vi "PIDController_AdvCalculate_FF_Sp_Pv.vi"(6 "Time":dbl=-1.0 format="%33.4f", 7 "Auto":bool=TRUE, 8 "FF":dbl, 9 "SP":dbl, 10 "PV":dbl, 11 "in PID_CONTROLLER":T1={"Kp"=0.0, "Ki"=0.0, "Kd"=0.0, "Period"=0.0, "Max_Integral"=0.0, "Min_Integral"=0.0, "Max_Input"=0.0, "Min_Input"=0.0, "Continuous"=FALSE, "PositionError"=0.0, "VelocityError"=0.0, "PrevError"=0.0, "TotalError"=0.0, "PositionTolerance"=0.0, "VelocityTolerance"=0.0, "SetPoint"=0.0, "Kf"=0.0, "Prev_Deriv"=0.0, "Prev_Deriv 2"=0.0, "DerivativeFilter"=FALSE, "Min_Output"=-9.99e+35, "Max_Output"=9.9e+35, "Prev_F_P"=0.0, "Prev_F_P_2"=0.0, "AntiWindupActive"=FALSE, "Measurement"=0.0} {"Measurement" format="%16_6e"; "Prev_F_P_2" format="%16_6e"; "Prev_F_P" format="%16_6e"; "Max_Output" format="%16_6e"; "Min_Output" format="%16_6e"; "Prev_Deriv 2" format="%16_6e"; "Prev_Deriv" format="%16_6e"; "Kf" format="%16_6e"; "SetPoint" format="%16_6e"; "VelocityTolerance" format="%16_6e"; "PositionTolerance" format="%16_6e"; "TotalError" format="%16_6e"; "PrevError" format="%16_6e"; "VelocityError" format="%16_6e"; "PositionError" format="%16_6e"; "Min_Input" format="%16_6e"; "Max_Input" format="%16_6e"; "Min_Integral" format="%16_6e"; "Max_Integral" format="%16_6e"; "Period" format="%16_6e"; "Kd" format="%16_6e"; "Ki" format="%16_6e"; "Kp" format="%16_6e"}) -> (1 "ControlOutput":dbl, 3 "out PID_CONTROLLER":T1={"Kp"=0.0, "Ki"=0.0, "Kd"=0.0, "Period"=0.0, "Max_Integral"=0.0, "Min_Integral"=0.0, "Max_Input"=0.0, "Min_Input"=0.0, "Continuous"=FALSE, "PositionError"=0.0, "VelocityError"=0.0, "PrevError"=0.0, "TotalError"=0.0, "PositionTolerance"=0.0, "VelocityTolerance"=0.0, "SetPoint"=0.0, "Kf"=0.0, "Prev_Deriv"=0.0, "Prev_Deriv 2"=0.0, "DerivativeFilter"=FALSE, "Min_Output"=-9.99e+35, "Max_Output"=9.9e+35, "Prev_F_P"=0.0, "Prev_F_P_2"=0.0, "AntiWindupActive"=FALSE, "Measurement"=0.0} {"Measurement" format="%16_6e"; "Prev_F_P_2" format="%16_6e"; "Prev_F_P" format="%16_6e"; "Max_Output" format="%16_6e"; "Min_Output" format="%16_6e"; "Prev_Deriv 2" format="%16_6e"; "Prev_Deriv" format="%16_6e"; "Kf" format="%16_6e"; "SetPoint" format="%16_6e"; "VelocityTolerance" format="%16_6e"; "PositionTolerance" format="%16_6e"; "TotalError" format="%16_6e"; "PrevError" format="%16_6e"; "VelocityError" format="%16_6e"; "PositionError" format="%16_6e"; "Min_Input" format="%16_6e"; "Max_Input" format="%16_6e"; "Min_Integral" format="%16_6e"; "Max_Integral" format="%16_6e"; "Period" format="%16_6e"; "Kd" format="%16_6e"; "Ki" format="%16_6e"; "Kp" format="%16_6e"})   [LabVIEW 2019, in "Trajectory_Library.lvlib"]
doc: "Returns the next output of the \"advanced\" PID controller. This controller implements the same PID as the \"normal\" controller with the following enhancements:\n - Integration by trapezoids is used.\n - Optionally filters derivative terms. (See SetDerivativeFilter subVI documentation for information.)\n - Incorporates optional feedforward.\n - Includes integral windup protection. This is only useful when output limits are specified.\n - When not called with a specific period, uses the actual elapsed time. (This subVI calculates the actual elapsed time.) \n - Limits the outputs. When output limits are specified the output is cooerced be within these limits.\n - Includes an Auto/Manual mode. In manual mode the scaled feedforward is sent directly to the output and the PID controller tracks this output value to allow for smooth transition back to auto mode.\n\nThe generalized equation for this PID when in auto is:\n CO = Kf x feedforward + Kp x error + Ki x Integral(error) + Kd x Derivative(error)\n\nWhen auto mode is disabled, the generaized equation is:\n CO = Kf x feedforward \n \nInputs:\n - PID_Controller -- PID_Controller data cluster\n - PV-measurement -- The current measurement of the process variable. (PV)\n - SP-setpoint -- The new setpoint of the controller. (SP)\n - FF-feedforward -- Feedforward n the same units as the PV and SP\n - Auto -- Use the PID calculate when this is True\n\nOutputs:\n - PID_Controller -- Updated PID_Controller data cluster\n - CO-ControlOutput -- Controller output (CO)"
uses:
  Trajectory_Library.lvlib
  TypeDef/PID_CONTROLLER.ctl
  PIDController_SetSetpoint.vi
  ControllerUtil_GetModulusError.vi
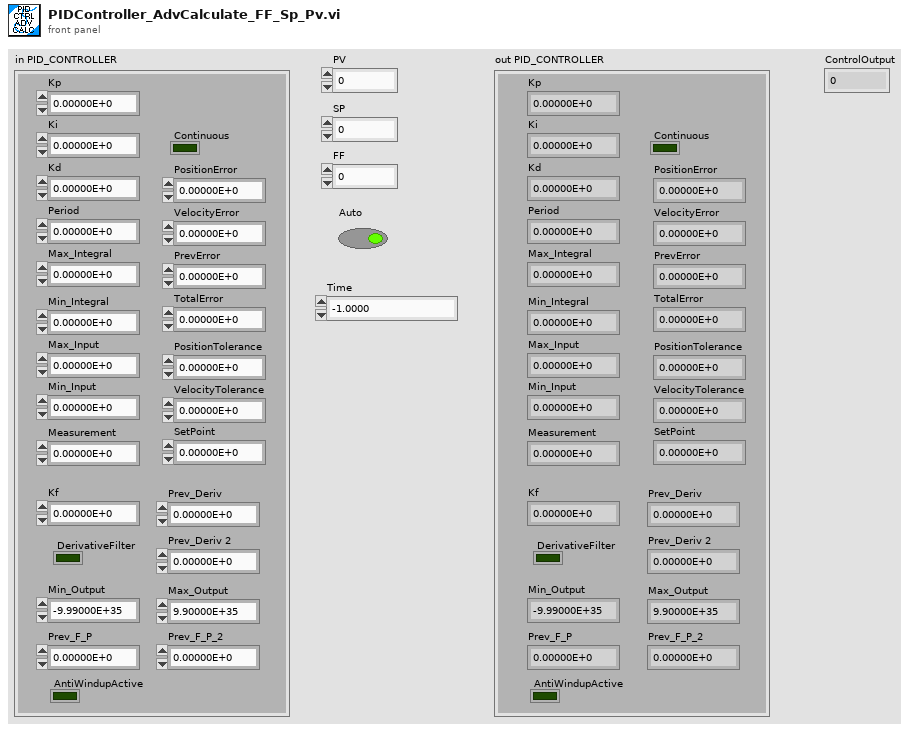
[diagram p1: front panel]
types:
  T1 = typedef "Trajectory_Library.lvlib/PID_CONTROLLER.ctl" = cluster{"Kp":dbl, "Ki":dbl, "Kd":dbl, "Period":dbl, "Max_Integral":dbl, "Min_Integral":dbl, "Max_Input":dbl, "Min_Input":dbl, "Continuous":bool, "PositionError":dbl, "VelocityError":dbl, "PrevError":dbl, "TotalError":dbl, "PositionTolerance":dbl, "VelocityTolerance":dbl, "SetPoint":dbl, "Kf":dbl, "Prev_Deriv":dbl, "Prev_Deriv 2":dbl, "DerivativeFilter":bool, "Min_Output":dbl, "Max_Output":dbl, "Prev_F_P":dbl, "Prev_F_P_2":dbl, "AntiWindupActive":bool, "Measurement":dbl}
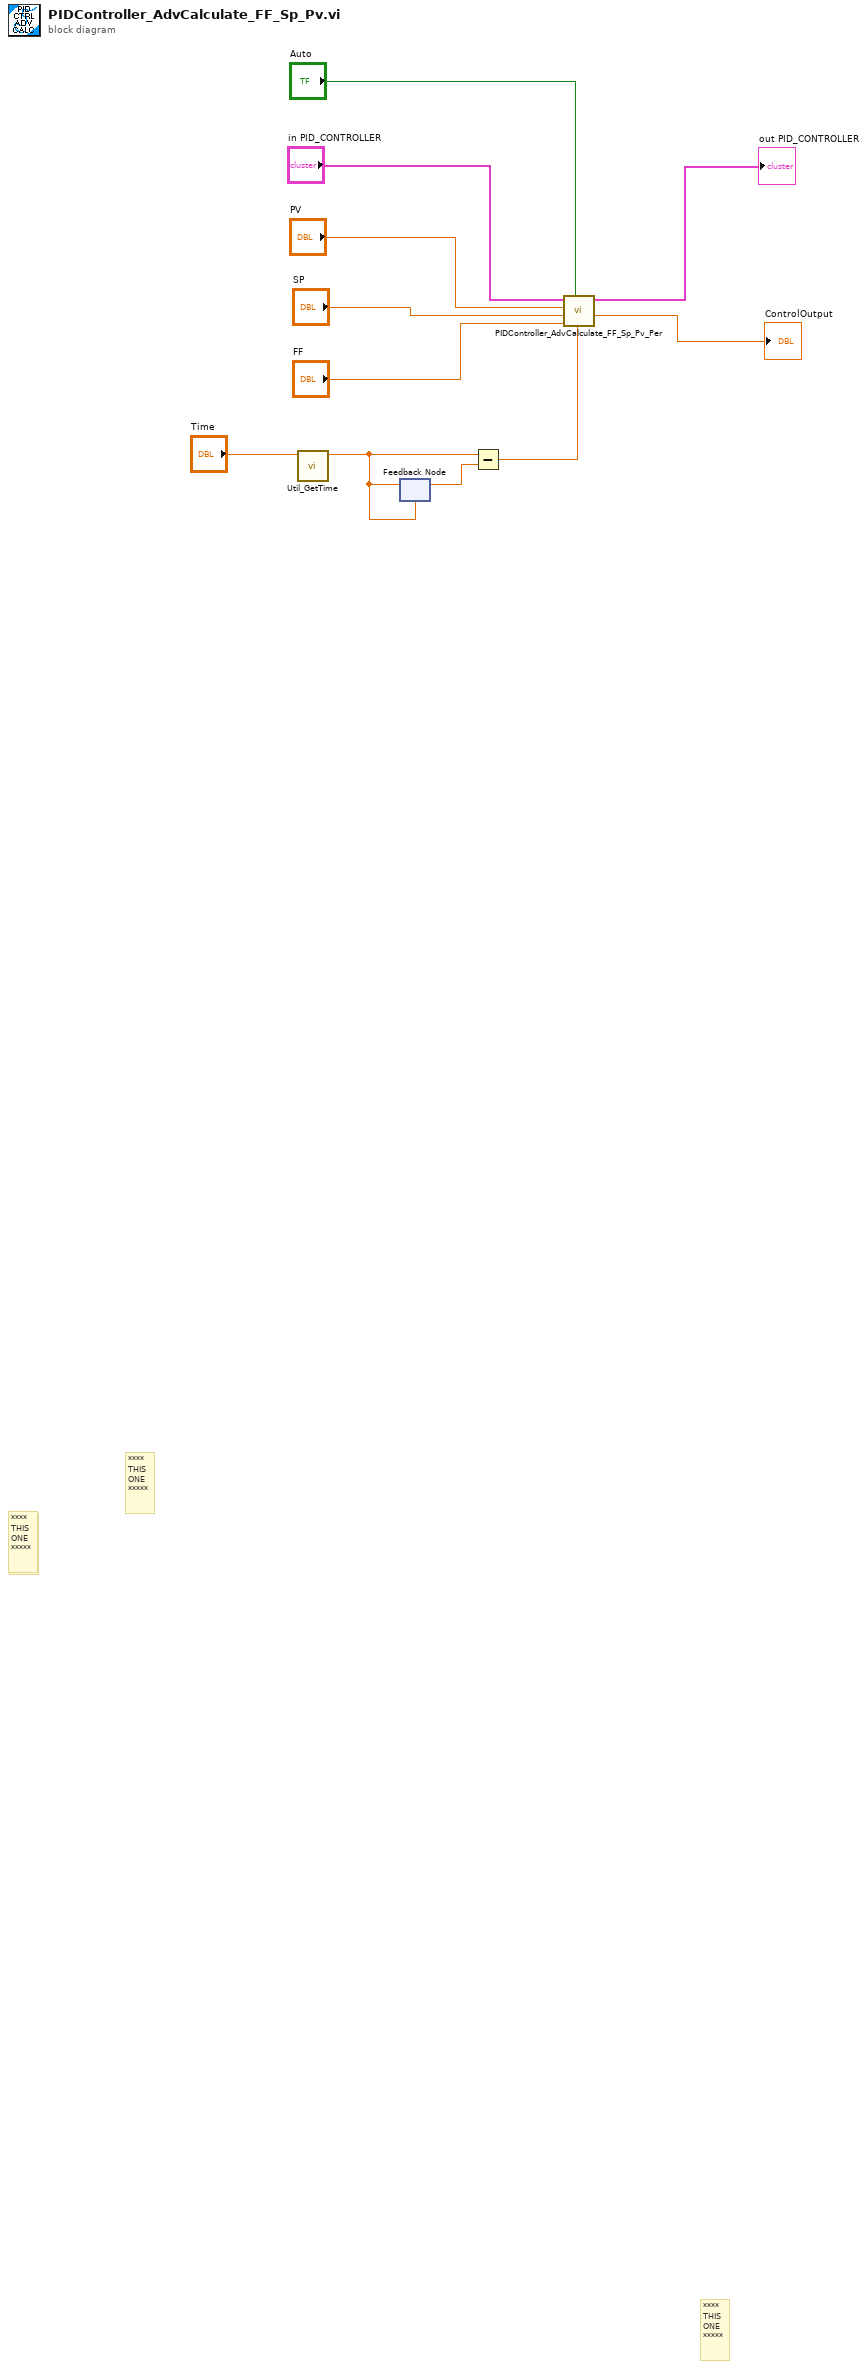
[diagram p0: block diagram]
diagram:
  # "****\nTHIS\nONE\n*****"
  # "****\nTHIS\nONE\n*****"
  # "****\nTHIS\nONE\n*****"
  # "****\nTHIS\nONE\n*****"
  n1 = call "Util_GetTime.vi"("Pass_Through_Time"="Time") -> ("FPGA_Time_Seconds"=w6:dbl)  [unwired: 9 in, 1 out]
  n2 = feedback-in #1(w6) -> ()
  n3 = feedback #1(w6) -> (w5:dbl)
  n4 = Subtract(x=w6, y=w5) -> (x-y=w4:dbl)
  n5 = call "PIDController_AdvCalculate_FF_Sp_Pv_Per.vi"("Period"=w4, "Auto"="Auto", "FF"="FF", "SP"="SP", "PV"="PV", "in PID_CONTROLLER"="in PID_CONTROLLER") -> ("ControlOutput"=→"ControlOutput":dbl, "out PID_CONTROLLER"=→"out PID_CONTROLLER":T1)  [unwired: 4 in]
